vi "cook.vi"(8 "error in (no error)":errorcluster, 11 "Phone in":refnum<class "Phone.lvclass">) -> (0 "error out":errorcluster, 3 "Phone out":refnum<class "Phone.lvclass">)   [LabVIEW 2011, in "Phone.lvclass"]
uses:
  Phone.lvclass
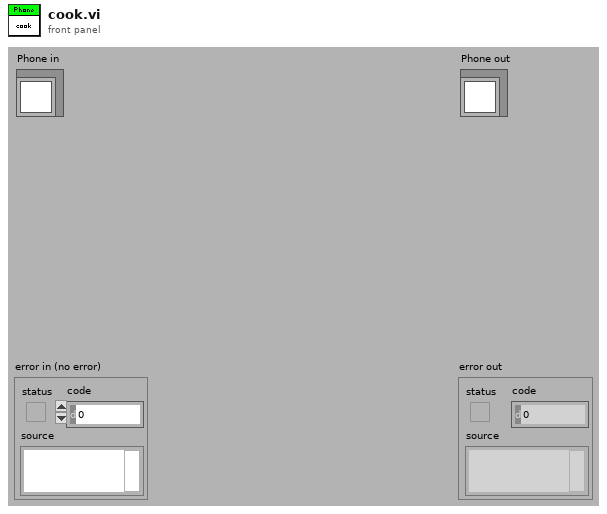
[diagram p1: front panel]
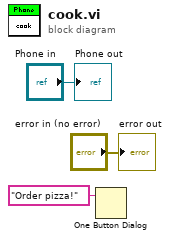
[diagram p0: block diagram]
diagram:
  n1 = One Button Dialog(message="Order pizza!") -> ()  [unwired: 1 in, 1 out]
  "error out" <- "error in (no error)"
  "Phone out" <- "Phone in"
